vi "Avantes - Determine Integration Time.vi"(6 "a_pSpectrum":dbl[](array[numeric]), 7 "a_pSaturated":u8[](array[numeric]), 8 "error in (no error)":errorcluster, 10 "Saturated?":bool, 11 "AVS Settings In":T1) -> (0 "error out":errorcluster, 1 "Continue Int Time Seek":bool=TRUE, 3 "AVS Settings Out":T1)   [LabVIEW 2013, in "AvaSpec.lvlib" / "AvaSpec Acquisition.lvlib"]
uses:
  AvaSpec Acquisition.lvlib
  Libraries/AS-5216-DLL/AVS settings.ctl
  AvaSpec.lvlib
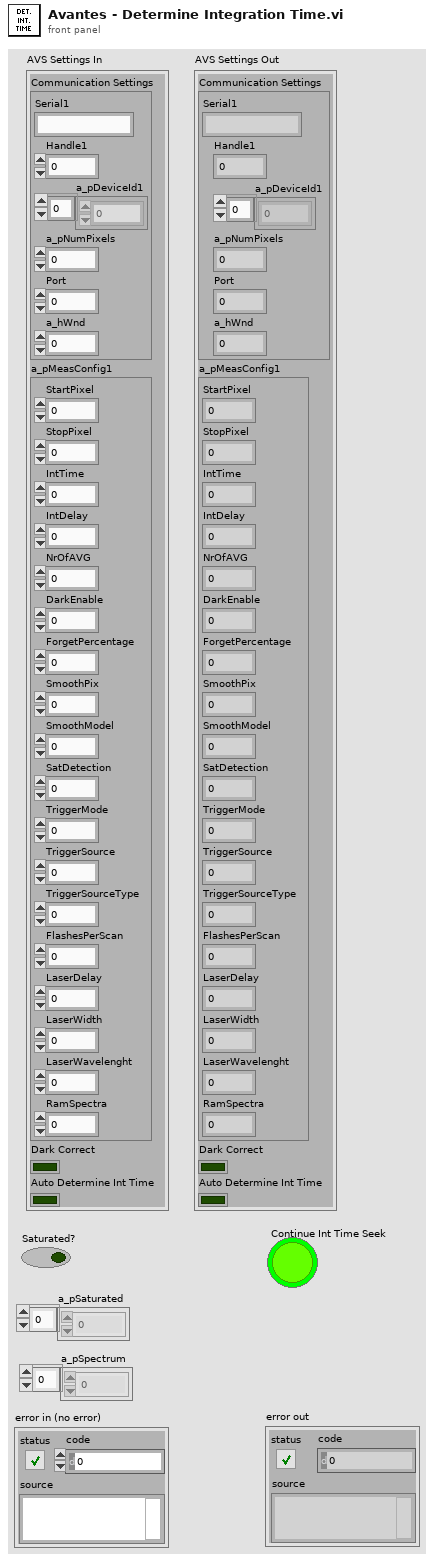
[diagram p1: front panel]
types:
  T1 = typedef "AvaSpec.lvlib/AVS settings.ctl" = cluster{"Communication Settings":cluster{"Serial1":string, "Handle1":i32, "a_pDeviceId1":u8[], "a_pNumPixels":u16, "Port":i32, "a_hWnd":i32}, "a_pMeasConfig1":cluster{"StartPixel":u16, "StopPixel":u16, "IntTime":sgl, "IntDelay":u32, "NrOfAVG":u32, "DarkEnable":u8, "ForgetPercentage":u8, "SmoothPix":u16, "SmoothModel":u8, "SatDetection":u8, "TriggerMode":u8, "TriggerSource":u8, "TriggerSourceType":u8, "FlashesPerScan":u16, "LaserDelay":u32, "LaserWidth":u32, "LaserWavelenght":sgl, "RamSpectra":u16}, "Dark Correct":bool, "Auto Determine Int Time":bool}
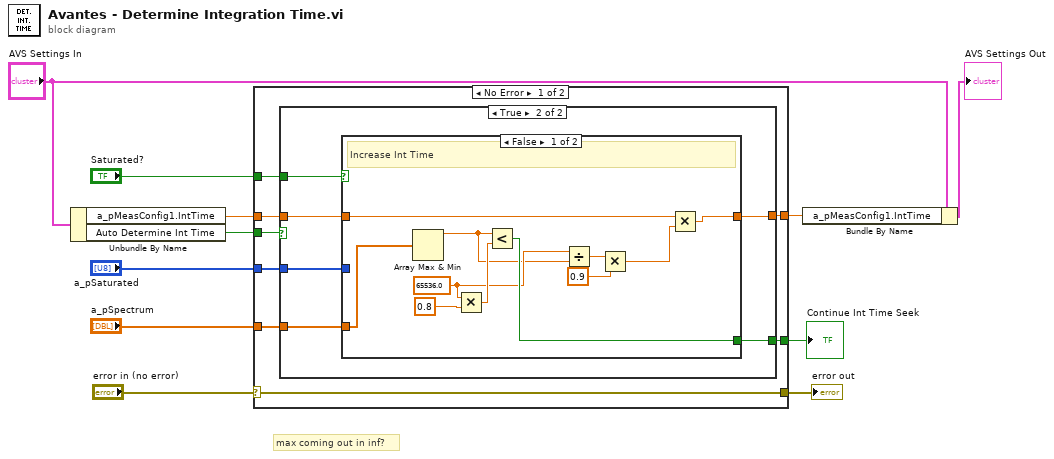
[diagram p0: block diagram]
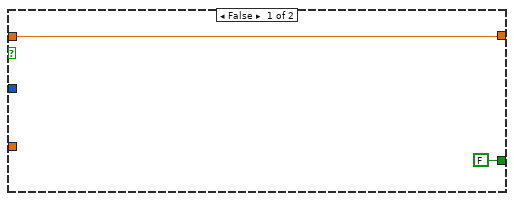
[diagram p2: hidden frame]
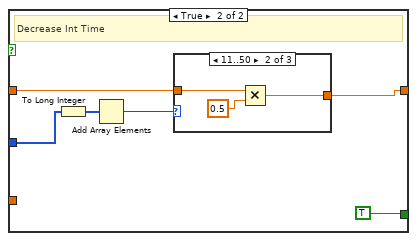
[diagram p3: hidden frame]
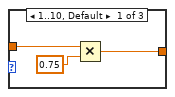
[diagram p4: hidden frame]
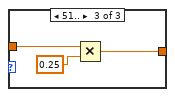
[diagram p5: hidden frame]
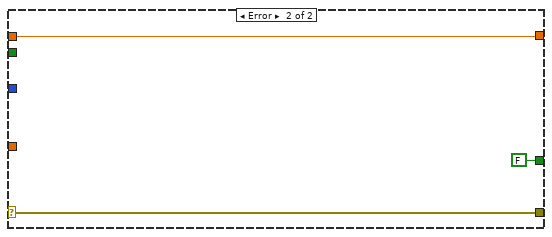
[diagram p6: hidden frame]
diagram:
  # "max coming out in inf?"
  n1 = Unbundle By Name("AVS Settings In") -> ("a_pMeasConfig1.IntTime"=w9:sgl, "Auto Determine Int Time"=w1:bool)
  n2 = case shown="No Error" "error in (no error)" {
    selector: "error in (no error)" -> [w13 w54]
    tunnel: [w19 w56] -> w11
    tunnel: "a_pSpectrum" -> [w18 _]
    tunnel: w9 -> [w17 w56]
    tunnel: "a_pSaturated" -> [w16 _]
    tunnel: [w15 FALSE] -> w7
    tunnel: "Saturated?" -> [w14 _]
    tunnel: [w13 w54] -> w2
    tunnel: w1 -> [w12 _]
    frame No Error {
      n3 = case shown="True" w12 {
        tunnel: [w20 w27] -> w19
        tunnel: w18 -> [_ w26]
        tunnel: w17 -> [w20 w25]
        tunnel: w16 -> [_ w24]
        tunnel: [FALSE w23] -> w15
        tunnel: w14 -> [_ w22]
        frame False {
        }
        frame True {
          n4 = case shown="False" w22 {
            tunnel: [w33 w39] -> w27
            tunnel: w26 -> [w36 _]
            tunnel: w25 -> [w34 w40]
            tunnel: w24 -> [_ w43]
            tunnel: [w35 TRUE] -> w23
            frame False {
              w32 = 65536.0
              # "Increase Int Time"
              n5 = Array Max & Min(array=w36) -> (max value=w31:dbl)  [unwired: 3 out]
              n6 = Multiply(x=w32, y=0.8) -> (x*y=w37:dbl)
              n7 = Less?(x=w31, y=w37) -> (x < y?=w35:bool)
              n8 = Divide(x=w32, y=w31) -> (x/y=w29:dbl)
              n9 = Multiply(x=w29, y=0.9) -> (x*y=w28:dbl)
              n10 = Multiply(x=w34, y=w28) -> (x*y=w33:dbl)
            }
            frame True {
              # "Decrease Int Time"
              n11 = To Long Integer(number=w43) -> (32bit integer=w44:i32[])
              n12 = Add Array Elements(numeric array=w44) -> (sum=w41:i32)
              n13 = case shown="11..50" w41 {
                tunnel: w40 -> [w47 w50 w53]
                tunnel: [w45 w48 w51] -> w39
                frame 1..10, Default {
                  n14 = Multiply(x=w47, y=sgl 0.75) -> (x*y=w45:sgl)
                }
                frame 11..50 {
                  n15 = Multiply(x=w50, y=sgl 0.5) -> (x*y=w48:sgl)
                }
                frame 51.. {
                  n16 = Multiply(x=w53, y=sgl 0.25) -> (x*y=w51:sgl)
                }
              }
            }
          }
        }
      }
    }
    frame Error {
    }
  }
  "Continue Int Time Seek" <- w7
  "error out" <- w2
  n17 = Bundle By Name(cluster="AVS Settings In", "a_pMeasConfig1.IntTime"=w11) -> (→"AVS Settings Out":T1)
